vi "readText.vi"(8 "error in (no error)":errorcluster, 11 "MS-Word in":refnum<class "MS-Word.lvclass">) -> (0 "error out":errorcluster, 2 "Text":string, 3 "MS-Word out":refnum<class "MS-Word.lvclass">)   [LabVIEW 2017, in "LabVIEW NPOI.lvlib" / "MS-Word.lvclass"]
uses:
  MS-Word.lvclass
  MS-Word.lvclass/MS-Word.ctl
  C:/Users/Neo/Desktop/Dev_Tools_BR/LabVIEW_NPOI/lib/NPOI 2.1.1/NPOI.OOXML.dll
  lib/NPOI 2.1.1/NPOI.OOXML.dll
panel:
  out "Text 2":string
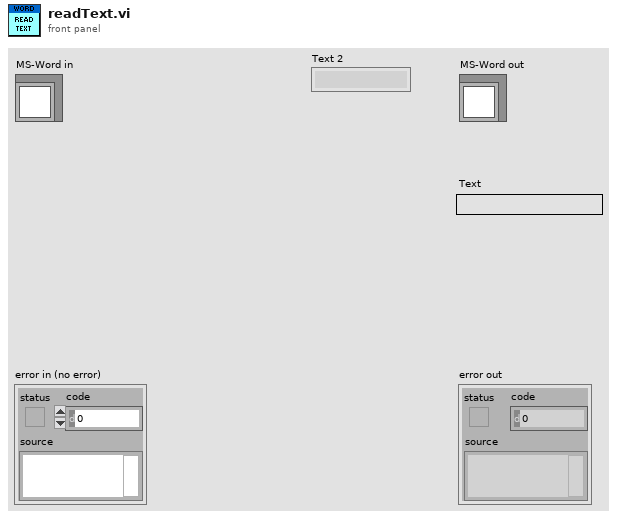
[diagram p1: front panel]
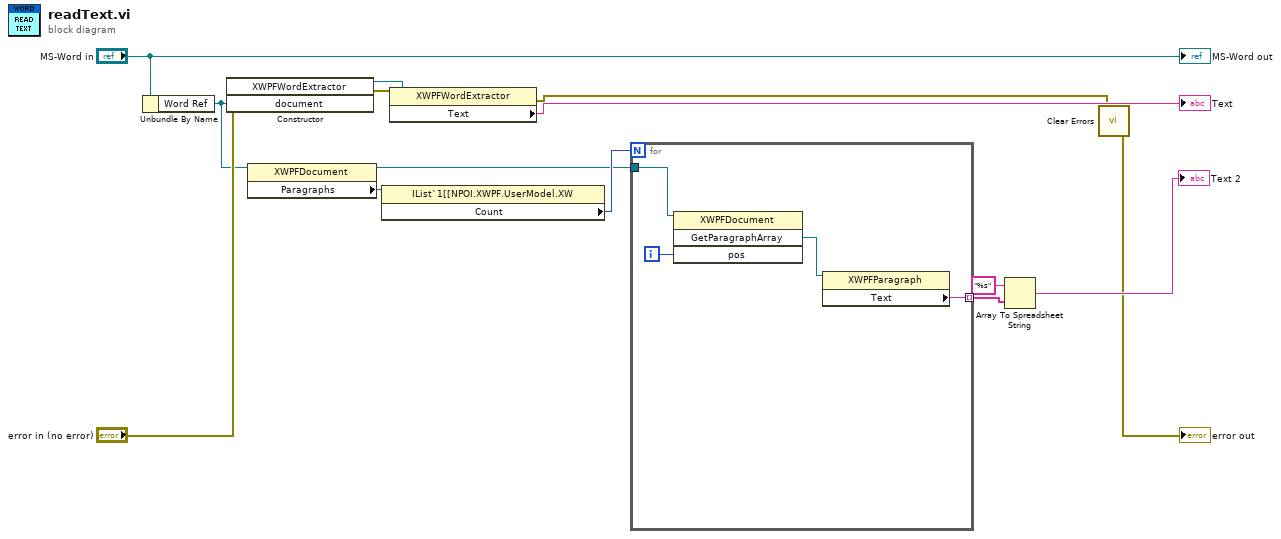
[diagram p0: block diagram]
diagram:
  n1 = Unbundle By Name("MS-Word in") -> ("Word Ref"=w8:refnum<k24>)
  n2 = constructor class="XWPFWordExtractor"(error in="error in (no error)", "document"=w8) -> (reference out=w10:refnum<k24>, error out=w13:errorcluster)  [unwired: 2 in, 2 out]
  n3 = property class="XWPFDocument"(reference=w8) -> (reference out=w5:refnum<k24>, "Paragraphs"=w7:refnum<k24>)  [unwired: 1 in, 1 out]
  n4 = property class="IList`1[[NPOI.XWPF.UserModel.XW"(reference=w7) -> ("Count"=w6:i32)  [unwired: 1 in, 2 out]
  n5 = property class="XWPFWordExtractor"(reference=w10, error in=w13) -> (error out=w9:errorcluster, "Text"=→"Text":string)  [unwired: 1 out]
  n6 = for {
    N: w6 -> [_]
    tunnel: w5 -> [w18]
    tunnel: [w15] -> w4 mode=indexing
    i -> [w17]
    n7 = invoke class="XWPFDocument" method="GetParagraphArray"(reference=w18, "pos"=w17) -> ("GetParagraphArray"=w16:refnum<k24>)  [unwired: 2 in, 3 out]
    n8 = property class="XWPFParagraph"(reference=w16) -> ("Text"=w15:string)  [unwired: 1 in, 2 out]
  }
  n9 = Array To Spreadsheet String(array=w4, 3:"%s" ("format string")) -> (spreadsheet string=→"Text 2":string)  [unwired: 1 in]
  n10 = call <vilib>:"Clear Errors.vi"("error in (no error)"=w9) -> ("error out"=→"error out":errorcluster)  [unwired: 5 in, 1 out]
  "MS-Word out" <- "MS-Word in"
